vi "Set Style Name.vi"(8 "error in (no error)":errorcluster, 10 "Style Name":string, 11 "Style in":refnum<class "Style.lvclass">) -> (0 "error out":errorcluster, 3 "Style out":refnum<class "Style.lvclass">)   [LabVIEW 2017, in "Styles.lvlib" / "Style.lvclass"]
uses:
  Style.lvclass
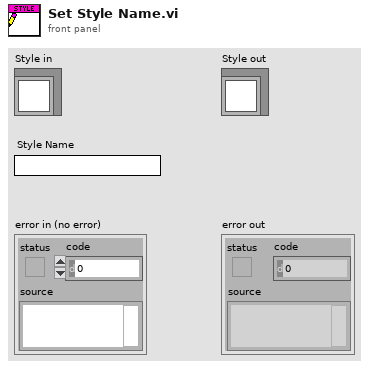
[diagram p1: front panel]
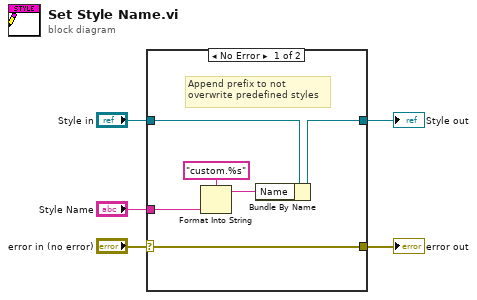
[diagram p0: block diagram]
diagram:
  n1 = case shown="No Error" "error in (no error)" {
    selector: "error in (no error)" -> [w11 w12]
    tunnel: [w11 w12] -> w4
    tunnel: [w9 w13] -> w2
    tunnel: "Style in" -> [w10 w13]
    tunnel: "Style Name" -> [w8 _]
    frame No Error {
      # "Append prefix to not\noverwrite predefined styles"
      n2 = Format Into String(format string="custom.%s", w8) -> (resulting string=w6:string)  [unwired: 2 in, 1 out]
      n3 = Bundle By Name(cluster=w10, "Name"=w6) -> (w9:refnum<class "Style.lvclass">)
    }
    frame Error {
    }
  }
  "error out" <- w4
  "Style out" <- w2
